vi "test-DiffDriveSim-XXX.vi"() -> ()   [LabVIEW 2019]
uses:
  <vilib>/Rock Robotics/WPI/ThirdParty/JAS_Junk/TrajLib/DCMOTOR.CTL
  <vilib>/Rock Robotics/WPI/ThirdParty/JAS_Junk/TrajLib/LINEAR_SYSTEM.ctl
  <vilib>/Analysis/Matrix/Datatypes/RealMatrix.ctl
  <vilib>/Rock Robotics/WPI/ThirdParty/JAS_Junk/TrajLib/LINEAR_QUADRATIC_REGULATOR.ctl
  <vilib>/Rock Robotics/WPI/ThirdParty/JAS_Junk/TrajLib/KALMAN_FILTER.ctl
  <vilib>/Rock Robotics/WPI/ThirdParty/JAS_Junk/TrajLib/LINEAR_SYSTEM_LOOP.ctl
  <vilib>/Rock Robotics/WPI/ThirdParty/JAS_Junk/TrajLib/LINEAR_PLANT_INV_FF.ctl
  <vilib>/Rock Robotics/WPI/ThirdParty/JAS_Junk/TrajLib/DIFF_DRIVE_TRAIN_SIM.ctl
  <vilib>/Rock Robotics/WPI/ThirdParty/JAS_Junk/TrajLib/DIFF_DRIVE_KitBot_WheelSize_ENUM.ctl
  <vilib>/Rock Robotics/WPI/ThirdParty/JAS_Junk/TrajLib/DIFF_DRIVE_ToughBoxMini_GearChoice_ENUM.ctl
  <vilib>/Rock Robotics/WPI/ThirdParty/JAS_Junk/TrajLib/DIFF_DRIVE_ToughBoxMini_MotorChoice_ENUM.ctl
  <vilib>/Rock Robotics/WPI/ThirdParty/JAS_Junk/TrajLib/DCMotor_New.vi
  <vilib>/Rock Robotics/WPI/ThirdParty/JAS_Junk/TrajLib/Units_RotationsPerMinuteToRadiansPerSecond.vi
  <vilib>/Rock Robotics/WPI/ThirdParty/JAS_Junk/TrajLib/MatBuilder_Create.vi
  <vilib>/Rock Robotics/WPI/ThirdParty/JAS_Junk/TrajLib/MatBuilder_Fill.vi
  <vilib>/Rock Robotics/WPI/ThirdParty/JAS_Junk/TrajLib/MatrixHelper_Zero.vi
  <vilib>/Rock Robotics/WPI/ThirdParty/JAS_Junk/TrajLib/LinearSystem_New.vi
  <vilib>/Rock Robotics/WPI/ThirdParty/JAS_Junk/TrajLib/Trajectory_Library.lvlib
  <vilib>/Analysis/Matrix/NI_Matrix.lvlib
panel:
  in  "Tab Control":T1(tab)
  in  "Arm Position\nRadians 2":dbl(slide) scale=-1.0..1.0
  out "Left Motor Vel (PV)":dbl format="%20.3f"
  out "Right Motor Vel (PV)":dbl format="%20.3f"
  out "Battery Voltage":dbl format="%20.3f"
  out "CO Chart":cluster{dbl, "Voltage":dbl}(graph)
  in  "Move Arm":bool
  out "Arm Position\nRadians":dbl(slide) scale=-1.0..4.0
  out "Cor Err":bool
  out "Kalman Filtered\nArm Angle":dbl format="%20.3f"
  out "PV Chart":T2(graph)
  out "Predict Err":bool
  out "Left Motor Volt Dmd (CO)":dbl format="%20.3f"
  out "Motor Amps":dbl format="%20.3f"
  out "Sim Upd Err":bool
  out "Right Motor Volt Dmd (CO)":dbl format="%20.3f"
  out "DiffDriveMotor":T3 {"Jr_KgM2" format="%13.5p"; "L_H" format="%13.5p"; "Kt_NMPerAmp" format="%13.5p"; "KvINV_RadPerSecPerVolt" format="%13.5p"; "R_Ohms" format="%13.5p"; "FreeSpeed_RadPerSec" format="%13.5p"; "FreeCurrent_Amps" format="%13.5p"; "StallCurrent_Amps" format="%13.5p"; "StallTorque_NM" format="%13.5p"; "nominalVoltage_Volts" format="%13.5p"}
  out "m_DiffDriveVel":T4
  out "Differential Drive Train Sim":T6 {"m_Motor"."Jr_KgM2" format="%13.5p"; "m_Motor"."L_H" format="%13.5p"; "m_Motor"."Kt_NMPerAmp" format="%13.5p"; "m_Motor"."KvINV_RadPerSecPerVolt" format="%13.5p"; "m_Motor"."R_Ohms" format="%13.5p"; "m_Motor"."FreeSpeed_RadPerSec" format="%13.5p"; "m_Motor"."FreeCurrent_Amps" format="%13.5p"; "m_Motor"."StallCurrent_Amps" format="%13.5p"; "m_Motor"."StallTorque_NM" format="%13.5p"; "m_Motor"."nominalVoltage_Volts" format="%13.5p"}
  out "KalmanFilter":T7
  out "Kalman Error":bool
  out "LinearQuadraticRegulator":T8
  out "LQR Error":bool
  out "Linear System Loop":T9
  out "LinSysLoop_Error":bool
  # "<States,States>"
  # "<States,Inputs>"
  # "<Outputs,States>"
  # "<Outputs,Inputs>"
  # "<States, 1>"
  # "<Outputs, 1>"
  # "<Inputs, 1>"
  # "<Outputs, 1>"
  # "<States,States>"
  # "<States,Inputs>"
  # "<Outputs,States>"
  # "<Outputs,Inputs>"
  # "Steady State Gain  \n<States,Outputs>"
  # "State Estimate <Statess,1>"
  # "<States,States>"
  # "<States,Inputs>"
  # "<Outputs,States>"
  # "<Outputs,Inputs>"
  # "Ref State <States,1>"
  # "Comp and capped \noutput <Inputs,1>"
  # "Controller gain\n<Inputs,States>"
  # "<States,1>"
  # "<FUTURE --- CLAMP TYPE -- For now\nuse Normalize>"
  # "Steady State Gain  \n<States,Outputs>"
  # "State Estimate <Statess,1>"
  # "<States,States>"
  # "<States,Inputs>"
  # "<Outputs,States>"
  # "<Outputs,Inputs>"
  # "<States,1>"
  # "<Inputs,1>"
  # "<States,Inputs>"
  # "<States,States>"
  # "Ref State <States,1>"
  # "Comp and capped \noutput <Inputs,1>"
  # "Controller gain\n<Inputs,States>"
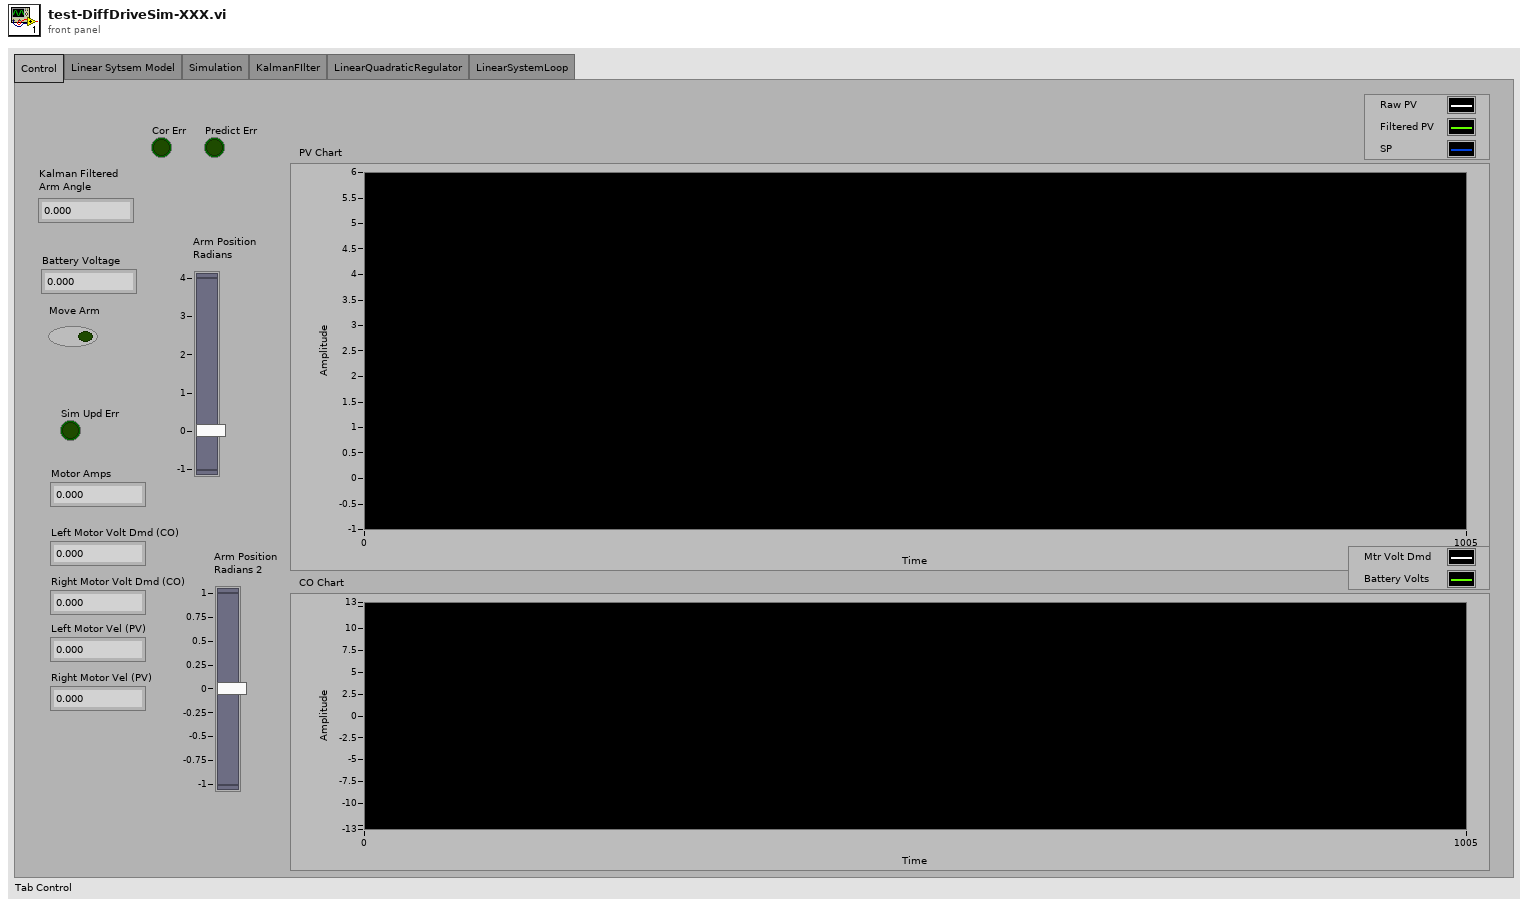
[diagram p1: front panel]
types:
  T1 = enum32{"Control", "Linear Sytsem Model", "Simulation", "KalmanFIlter", "LinearQuadraticRegulator", "LinearSystemLoop"}
  T2 = cluster{"upper limit":dbl, "Real Matrix Element":dbl, "Real Matrix Element":dbl}
  T3 = typedef "Trajectory_Library.lvlib/DCMOTOR.CTL" = cluster{"nominalVoltage_Volts":dbl, "StallTorque_NM":dbl, "StallCurrent_Amps":dbl, "FreeCurrent_Amps":dbl, "FreeSpeed_RadPerSec":dbl, "R_Ohms":dbl, "KvINV_RadPerSecPerVolt":dbl, "Kt_NMPerAmp":dbl, "L_H":dbl, "Jr_KgM2":dbl}
  T4 = typedef "Trajectory_Library.lvlib/LINEAR_SYSTEM.ctl" = cluster{"m_A":T5, "m_B":T5, "m_C":T5, "m_D":T5, "States":i32, "Inputs":i32, "Outputs":i32}
  T5 = typedef "NI_Matrix.lvlib/RealMatrix.ctl" = dbl[][]
  T6 = typedef "Trajectory_Library.lvlib/DIFF_DRIVE_TRAIN_SIM.ctl" = cluster{"m_Plant":T4, "m_X":T5, "m_Y":T5, "m_U":T5, "MeasureStdDev":T5, "m_Motor":T3, "m_OriginalGearing":dbl, "m_CurrentGearing":dbl, "m_WheelRadius_M":dbl, "m_RB":dbl}
  T7 = typedef "Trajectory_Library.lvlib/KALMAN_FILTER.ctl" = cluster{"m_K":T5, "m_xHat":T5, "States":i32, "Outputs":i32, "m_Plant":T4}
  T8 = typedef "Trajectory_Library.lvlib/LINEAR_QUADRATIC_REGULATOR.ctl" = cluster{"m_r":T5, "m_U":T5, "m_K":T5, "States":i32, "Inputs":i32}
  T9 = typedef "Trajectory_Library.lvlib/LINEAR_SYSTEM_LOOP.ctl" = cluster{"Controller":T8, "FeedForward":T10, "Observer":T7, "Next_R":T5, "Clamp Max":T5}
  T10 = typedef "Trajectory_Library.lvlib/LINEAR_PLANT_INV_FF.ctl" = cluster{"m_R":T5, "m_Uff":T5, "m_B":T5, "m_A":T5, "States":i32, "Inputs":i32}
  T11 = typedef "Trajectory_Library.lvlib/DIFF_DRIVE_ToughBoxMini_MotorChoice_ENUM.ctl" = enum16{"One CIM Per Side", "Two CIM Per Side", "One MiniCIM Per Side", "Two Mini CIM Per Side", "Two Falcon Per Side", "Two NEO Per Side"}
  T12 = typedef "Trajectory_Library.lvlib/DIFF_DRIVE_ToughBoxMini_GearChoice_ENUM.ctl" = enum16{"Ratio_12_75", "Ratio_10_71", "Ratio_8_45", "Ratio_7_31", "Ratio_5_95"}
  T13 = typedef "Trajectory_Library.lvlib/DIFF_DRIVE_KitBot_WheelSize_ENUM.ctl" = enum16{"4 Inch", "6 Inch", "8 Inch", "10 Inch"}
  T14 = cluster{"LeftVelocity_M_Per_Sec":dbl, "Real Matrix Element":dbl, "Real Matrix Element":dbl}
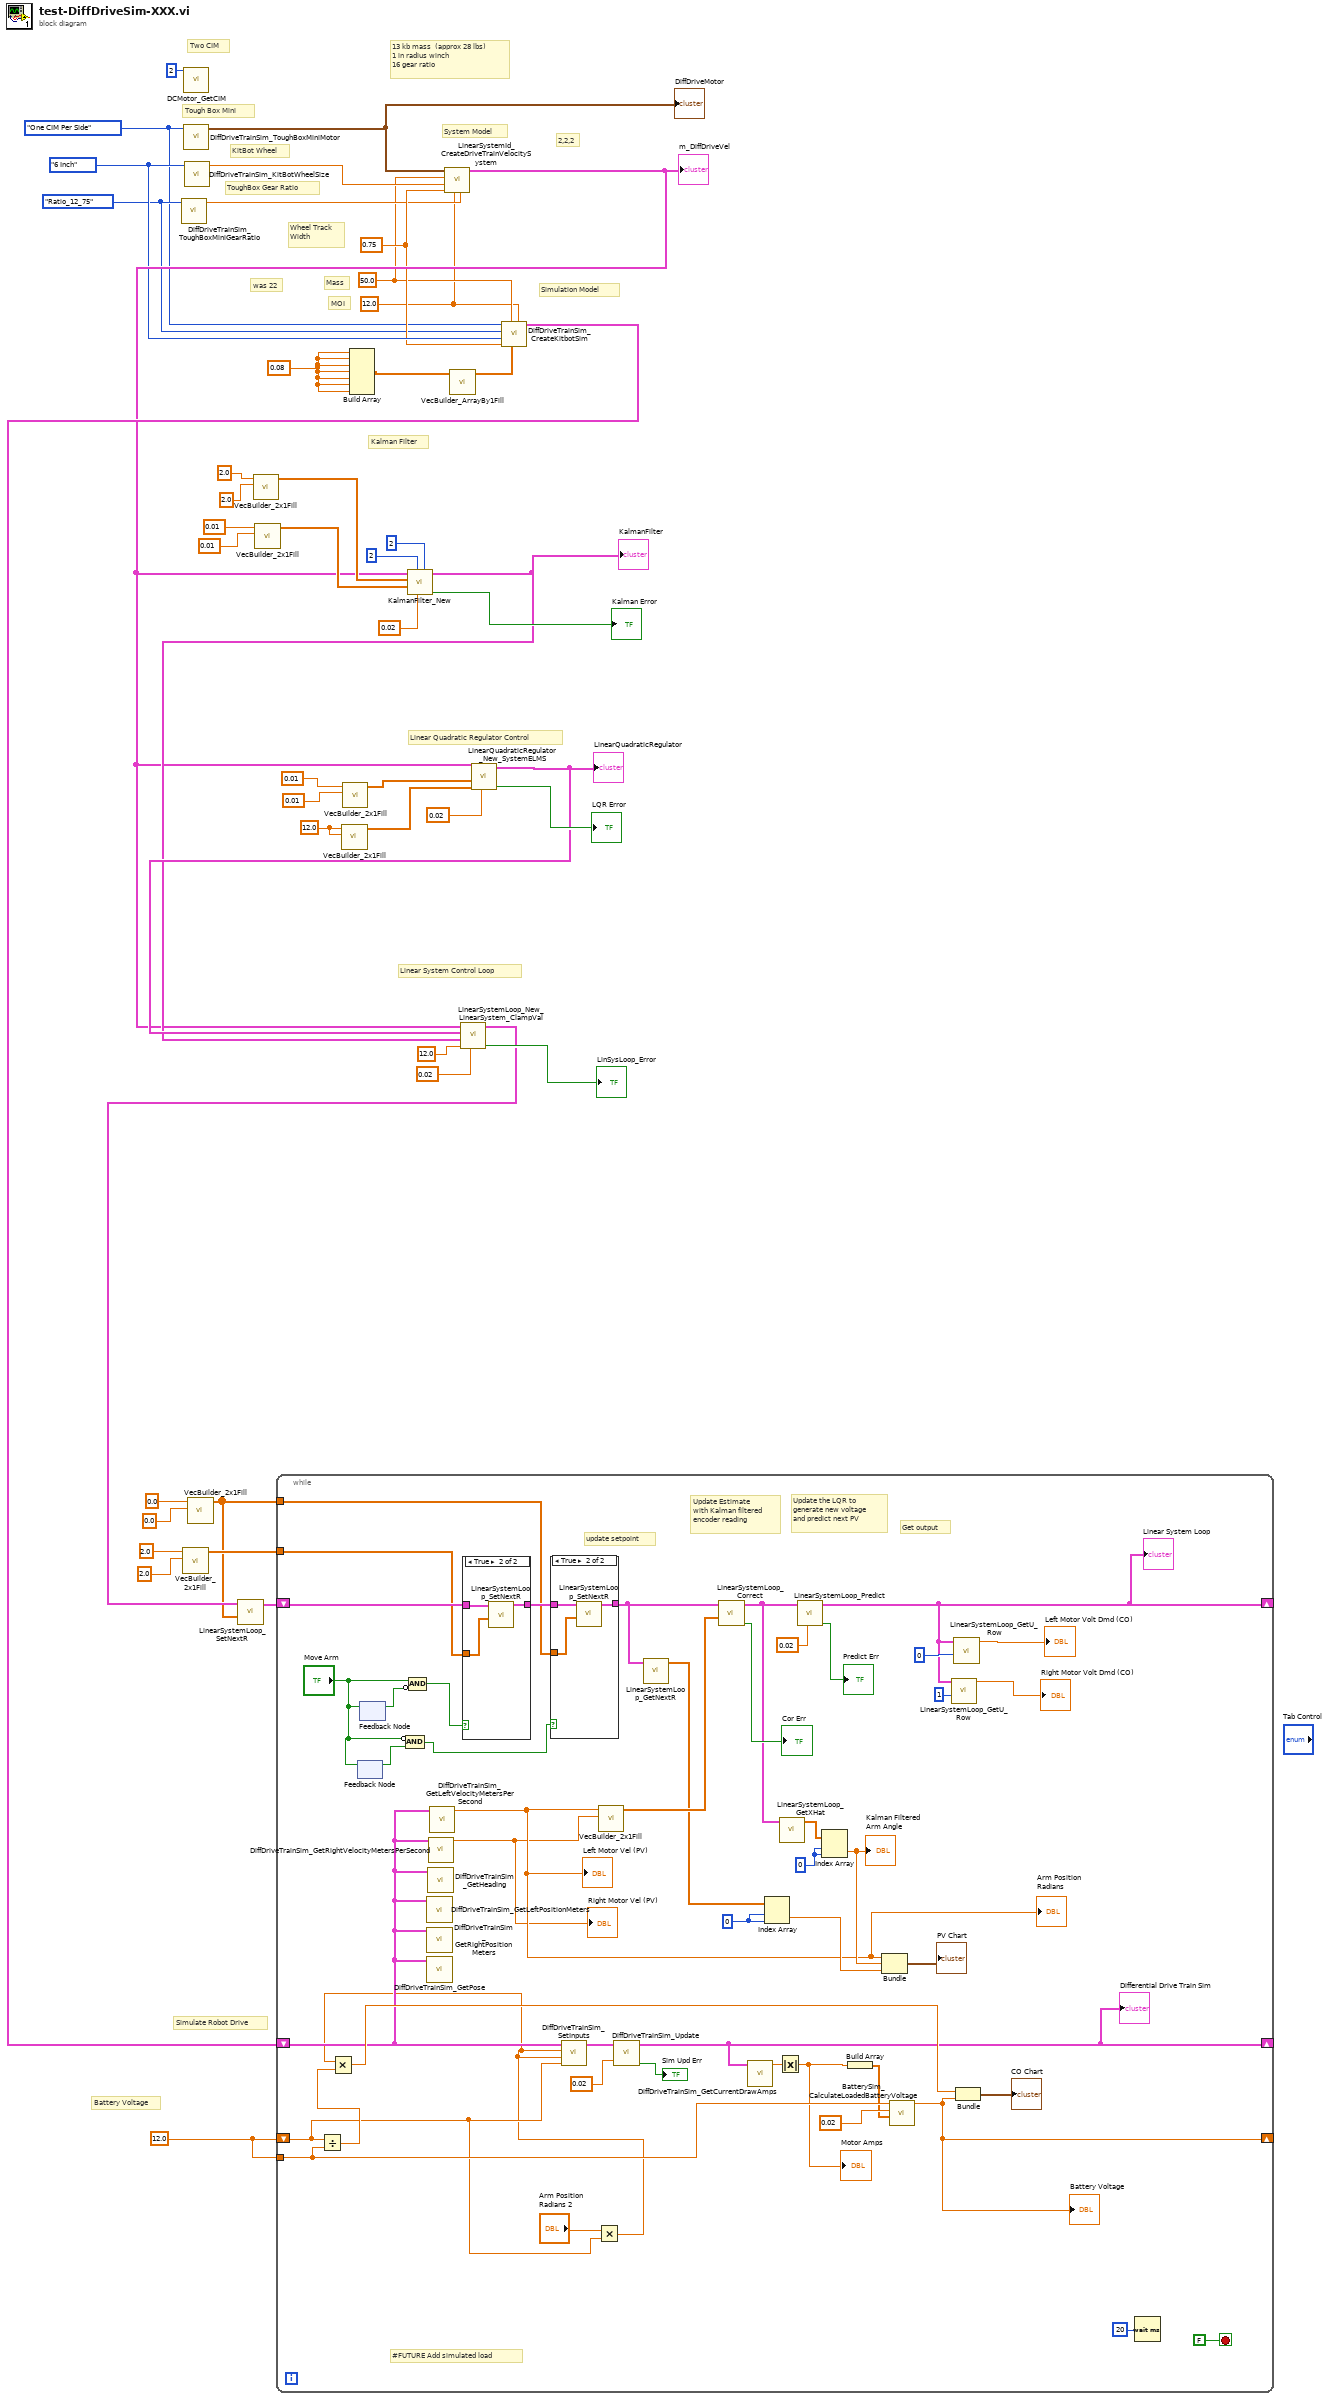
[diagram p0: block diagram]
diagram:
  w8 = 12.0 ("Mass_Kg")
  w9 = DIFF_DRIVE_ToughBoxMini_MotorChoice_ENUM."One CIM Per Side" ("ToughBoxMiniMotor")
  w11 = DIFF_DRIVE_ToughBoxMini_GearChoice_ENUM."Ratio_12_75" ("ToughBoxMiniGear")
  w15 = DIFF_DRIVE_KitBot_WheelSize_ENUM."6 Inch" ("Wheel Size")
  w10 = 50.0 ("Mass_Kg")
  w13 = 0.75 ("ArmLength_M")
  w4 = 12.0 ("R0_C0")
  w40 = 12.0
  w2 = 0.08 ("R0_C0")
  # "was 22"
  # "ToughBox Gear Ratio"
  # "KitBot Wheel"
  # "Tough Box Mini"
  # "Two CIM"
  # "2,2,2"
  # "MOI"
  # "Wheel Track\nWidth"
  # "Simulation Model"
  # "System Model"
  # "Mass"
  # "Kalman Filter"
  # "Linear Quadratic Regulator Control"
  # "Linear System Control Loop"
  # "Simulate Robot Drive"
  # "13 kb mass  (approx 28 lbs)\n1 in radius winch\n16 gear ratio"
  # "Battery Voltage"
  n1 = call <vilib>:"DiffDriveTrainSim_ToughBoxMiniGearRatio.vi"("ToughBoxMiniGear"=w11) -> ("GearRatio"=w12:dbl)  [unwired: 10 in]
  n2 = call <vilib>:"VecBuilder_2x1Fill.vi"("R1"=2.0, "R0"=2.0 ("RotationsPerMinute")) -> ("output matrix"=w24:T5)  [unwired: 9 in]
  n3 = call <vilib>:"DCMotor_GetCIM.vi"("Num Motors"=2) -> ()  [unwired: 10 in, 1 out]
  n4 = call <vilib>:"DiffDriveTrainSim_ToughBoxMiniMotor.vi"("ToughBoxMiniMotor"=w9) -> ("DriveMotor"=w1:T3)  [unwired: 10 in]
  "DiffDriveMotor" <- w1
  n5 = call <vilib>:"DiffDriveTrainSim_KitBotWheelSize.vi"("Wheel Size"=w15) -> ("WheelDiameter_M"=w16:dbl)  [unwired: 10 in]
  n6 = call <vilib>:"VecBuilder_2x1Fill.vi"("R1"=0.0, "R0"=0.0 ("R0_C0")) -> ("output matrix"=w18:T5)  [unwired: 9 in]
  n7 = call <vilib>:"VecBuilder_2x1Fill.vi"("R1"=2.0, "R0"=2.0 ("R0_C0")) -> ("output matrix"=w34:T5)  [unwired: 9 in]
  n8 = call <vilib>:"VecBuilder_2x1Fill.vi"("R1"=0.01, "R0"=0.01 ("R0_C0")) -> ("output matrix"=w33:T5)  [unwired: 9 in]
  n9 = call <vilib>:"VecBuilder_2x1Fill.vi"("R1"=w4, "R0"=w4) -> ("output matrix"=w28:T5)  [unwired: 9 in]
  n10 = call <vilib>:"VecBuilder_2x1Fill.vi"("R1"=0.01 ("R0_C0"), "R0"=0.01 ("R0_C0")) -> ("output matrix"=w30:T5)  [unwired: 9 in]
  n11 = Build Array(w2, w2, w2, w2, w2, w2, w2) -> (w3:dbl[])
  n12 = call <vilib>:"LinearSystemId_CreateDriveTrainVelocitySystem.vi"("G"=w12, "JKgMetersSquared"=w8, "rbMeters"=w13, "rMeters"=w16, "MassKg"=w10, "Motor"=w1) -> ("Linearsystem"=w17:T4)  [unwired: 4 in, 1 out]
  "m_DiffDriveVel" <- w17
  n13 = call <vilib>:"KalmanFilter_New.vi"("States"=2, "dt_Seconds"=0.02, "Outputs"=2, "MeasurementStdDevs"=w33, "StateStdDevs"=w34, "Plant"=w17) -> ("Error"=→"Kalman Error":bool, "KalmanFilter"=w43:T7)  [unwired: 4 in]
  "KalmanFilter" <- w43
  n14 = call <vilib>:"VecBuilder_ArrayBy1Fill.vi"("R Array"=w3) -> ("Output Vector"=w14:T5)  [unwired: 10 in]
  n15 = call <vilib>:"LinearQuadraticRegulator_New_SystemELMS.vi"("dt_Seconds"=0.02, "Relms"=w28, "Qelms"=w30, "LINEARSYSTEM"=w17) -> ("Error"=→"LQR Error":bool, "LinearQuadraticRegulator"=w44:T8)  [unwired: 6 in]
  "LinearQuadraticRegulator" <- w44
  n16 = call <vilib>:"LinearSystemLoop_New_LinearSystem_ClampVal.vi"("dT_Seconds"=0.02, "Max_Voltage"=12.0, "Observer"=w43, "Controller"=w44, "Plant"=w17) -> ("Error"=→"LinSysLoop_Error":bool, "Linear System Loop"=w20:T9)  [unwired: 5 in]
  n17 = call <vilib>:"LinearSystemLoop_SetNextR.vi"("R"=w18, "input inear System Loop"=w20) -> ("out Linear System Loop"=w21:T9)  [unwired: 8 in, 1 out]
  n18 = call <vilib>:"DiffDriveTrainSim_CreateKitbotSim.vi"("j_KgM2"=w8, "MeasurementStdDev"=w14, "Mass_Kg"=w10, "TrackWidth_M"=w13, "Wheelsize"=w15, "ToughBoxMiniGear"=w11, "ToughBoxMiniMotor"=w9) -> ("DiffDriveTrainSim"=w19:T6)  [unwired: 3 in, 1 out]
  n19 = while {
    shift-right: [w53] -> _
    shift-left: w21 -> [w65]
    tunnel: w24 -> [w63]
    tunnel: w18 -> [w64]
    shift-right: [w52] -> _
    shift-left: w19 -> [w57]
    shift-right: [w70] -> _
    shift-left: w40 -> [w48]
    tunnel: w40 -> [w74]
    stop <- FALSE stop-if-true
    w77 = 0 ("index (row)")
    w87 = 0 ("index (row)")
    # "#FUTURE Add simulated load"
    # "Get output"
    # "Update the LQR to \ngenerate new voltage\nand predict next PV"
    # "update setpoint"
    # "Update Estimate\nwith Kalman filtered\nencoder reading"
    n20 = Divide(x=w48, y=w74) -> (x/y=w75:dbl)
    n21 = feedback #1() -> (w91:bool)  [unwired: 1 in]
    n22 = feedback-in #1("Move Arm") -> ()
    n23 = feedback-in #2("Move Arm") -> ()
    n24 = feedback #2() -> (w92:bool)  [unwired: 1 in]
    n25 = Compound Arithmetic op=AND(invert "Move Arm", w91) -> (w61:bool)
    n26 = Compound Arithmetic op=AND("Move Arm", invert w92) -> (w62:bool)
    n27 = call <vilib>:"DiffDriveTrainSim_GetLeftPositionMeters.vi"("DiffDriveTrainSim"=w57) -> ()  [unwired: 10 in, 1 out]
    n28 = call <vilib>:"DiffDriveTrainSim_GetRightPositionMeters.vi"("DiffDriveTrainSim"=w57) -> ()  [unwired: 10 in, 1 out]
    n29 = call <vilib>:"DiffDriveTrainSim_GetPose.vi"("DiffDriveTrainSim"=w57) -> ()  [unwired: 10 in, 1 out]
    n30 = call <vilib>:"DiffDriveTrainSim_GetHeading.vi"("DiffDriveTrainSim"=w57) -> ()  [unwired: 10 in, 1 out]
    n31 = call <vilib>:"DiffDriveTrainSim_GetRightVelocityMetersPerSecond.vi"("DiffDriveTrainSim"=w57) -> ("RightVel_M_Per_Sec"=w50:dbl)  [unwired: 10 in]
    "Right Motor Vel (PV)" <- w50
    n32 = call <vilib>:"DiffDriveTrainSim_GetLeftVelocityMetersPerSecond.vi"("DiffDriveTrainSim"=w57) -> ("LeftVelocity_M_Per_Sec"=w51:dbl)  [unwired: 10 in]
    "Arm Position\nRadians" <- w51
    "Left Motor Vel (PV)" <- w51
    n33 = case shown="True" w62 {
      tunnel: [w95 w98] -> w66
      tunnel: w65 -> [w95 w97]
      tunnel: w63 -> [_ w96]
      frame False {
      }
      frame True {
        n34 = call <vilib>:"LinearSystemLoop_SetNextR.vi"("R"=w96, "input inear System Loop"=w97) -> ("out Linear System Loop"=w98:T9)  [unwired: 8 in, 1 out]
      }
    }
    n35 = case shown="True" w61 {
      tunnel: [w99 w102] -> w60
      tunnel: w66 -> [w99 w101]
      tunnel: w64 -> [_ w100]
      frame False {
      }
      frame True {
        n36 = call <vilib>:"LinearSystemLoop_SetNextR.vi"("R"=w100, "input inear System Loop"=w101) -> ("out Linear System Loop"=w102:T9)  [unwired: 8 in, 1 out]
      }
    }
    n37 = Multiply(x="Arm Position\nRadians 2", y=w48) -> (x*y=w47:dbl)
    n38 = Multiply(x=w47, y=w75) -> (x*y=w69:dbl)
    n39 = call <vilib>:"DiffDriveTrainSim_SetInputs.vi"("BatteryVoltage"=w48, "Right_Volts"=w47, "Left_Volts"=w47, "in DiffDriveTrainSim"=w57) -> ("out DiffDriveTrainSim"=w79:T6)  [unwired: 6 in, 1 out]
    n40 = call <vilib>:"VecBuilder_2x1Fill.vi"("R1"=w50, "R0"=w51) -> ("output matrix"=w89:T5)  [unwired: 9 in]
    n41 = call <vilib>:"DiffDriveTrainSim_Update.vi"("dT_Seconds"=0.02, "in DiffDriveTrainSim"=w79) -> ("Error"=→"Sim Upd Err":bool, "out DiffDriveTrainSim"=w52:T6)  [unwired: 8 in]
    "Differential Drive Train Sim" <- w52
    n42 = call <vilib>:"LinearSystemLoop_GetNextR.vi"("input inear System Loop"=w60) -> ("NextR"=w59:T5)  [unwired: 10 in]
    n43 = call <vilib>:"LinearSystemLoop_Correct.vi"("Y"=w89, "input inear System Loop"=w60) -> ("Error"=→"Cor Err":bool, "out Linear System Loop"=w83:T9)  [unwired: 8 in]
    n44 = call <vilib>:"DiffDriveTrainSim_GetCurrentDrawAmps.vi"("DiffDriveTrainSim"=w52) -> ("TotalCurrent_Amps"=w68:dbl)  [unwired: 10 in]
    n45 = Index Array(array=w59, index (row)=w77, index (col)=w77) -> (element=w76:dbl)
    n46 = Absolute Value(x=w68) -> (abs(x)=w67:dbl)
    "Motor Amps" <- w67
    n47 = call <vilib>:"LinearSystemLoop_GetXHat.vi"("input inear System Loop"=w83) -> ("XHat"=w86:T5)  [unwired: 10 in]
    n48 = call <vilib>:"LinearSystemLoop_Predict.vi"("dT_Seconds"=0.02, "input inear System Loop"=w83) -> ("Error"=→"Predict Err":bool, "out Linear System Loop"=w53:T9)  [unwired: 8 in]
    "Linear System Loop" <- w53
    n49 = Index Array(array=w86, index (row)=w87, index (col)=w87) -> (element=w85:dbl)
    "Kalman Filtered\nArm Angle" <- w85
    n50 = Build Array(w67) -> (w72:dbl[])
    n51 = Bundle("LeftVelocity_M_Per_Sec"=w51, "Real Matrix Element"=w85, "Real Matrix Element"=w76) -> (→"PV Chart":T14)  [unwired: 1 in]
    n52 = call <vilib>:"BatterySim_CalculateLoadedBatteryVoltage.vi"("Currents"=w72, "Resistance_Ohms"=0.02, "NominalVoltage"=w74) -> ("Voltage"=w70:dbl)  [unwired: 8 in]
    "Battery Voltage" <- w70
    n53 = call <vilib>:"LinearSystemLoop_GetU_Row.vi"("Row"=1, "input inear System Loop"=w53) -> ("U"=→"Right Motor Volt Dmd (CO)":dbl)  [unwired: 9 in]
    n54 = call <vilib>:"LinearSystemLoop_GetU_Row.vi"("Row"=0, "input inear System Loop"=w53) -> ("U"=→"Left Motor Volt Dmd (CO)":dbl)  [unwired: 9 in]
    n55 = Bundle(w69, "Voltage"=w70) -> (→"CO Chart":cluster{dbl, "Voltage":dbl})  [unwired: 1 in]
    n56 = Wait (ms)(milliseconds to wait=u32 20) -> ()  [unwired: 1 out]
  }
